vi "Variant to JSON String.vi"(6 "enable LabVIEW extensions? (T)":bool=TRUE, 7 "pretty print? (F)":bool, 8 "error in (no error)":errorcluster, 11 "Variant in":variant) -> (0 "error out":errorcluster, 2 "String":string, 3 "Variant out":variant)   [LabVIEW 2020, in "Variant JSON API.lvlib"]
uses:
  Variant JSON API.lvlib
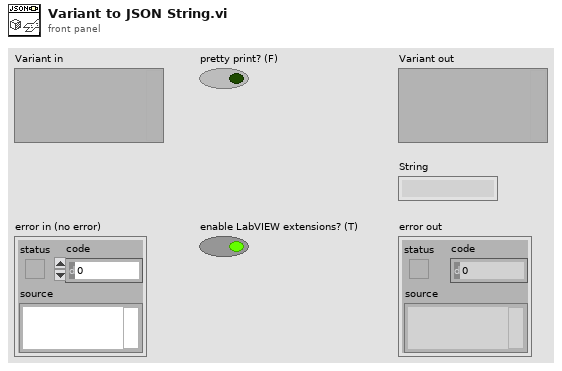
[diagram p1: front panel]
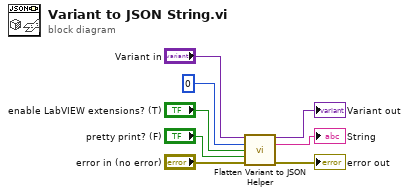
[diagram p0: block diagram]
diagram:
  n1 = call "Flatten Variant to JSON Helper.vi"("Variant in"="Variant in", "indent"=0, "enable LabVIEW extensions? (T)"="enable LabVIEW extensions? (T)", "pretty print? (T)"="pretty print? (F)", "error in (no error)"="error in (no error)") -> ("Variant out"=→"Variant out":variant, "String"=→"String":string, "error out"=→"error out":errorcluster)  [unwired: 8 in]
